vi "Linear to dB (scalar).vi"(1 "Linear":dbl) -> (0 "dB":dbl)   [LabVIEW 2020]
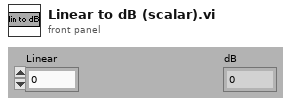
[diagram p1: front panel]
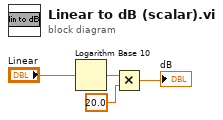
[diagram p0: block diagram]
diagram:
  n1 = Logarithm Base 10(1:"Linear") -> (0:w4:dbl)
  n2 = Multiply(x=w4, y=20.0) -> (x*y=→"dB":dbl)
